vi "Query.vi"(7 "Module Settings":T1(array[cluster]), 8 "error in (no error)":errorcluster, 9 "Region":dbl, 10 "Tray":dbl, 11 "Database Assembly in":refnum<class "Database Assembly.lvclass">) -> (0 "error out":errorcluster, 3 "Database Assembly out":refnum<class "Database Assembly.lvclass">)   [LabVIEW 2018, in "Database Assembly.lvclass"]
uses:
  Database Assembly.lvclass
  Module/Module.lvclass
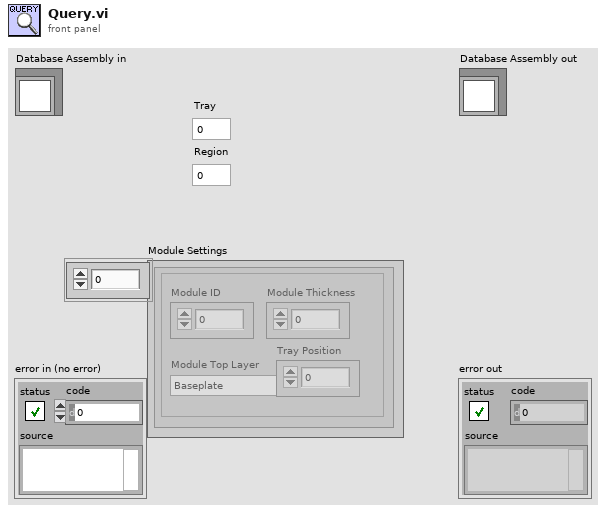
[diagram p1: front panel]
types:
  T1 = cluster{"Module ID":dbl, "Module Thickness":dbl, "Module Top Layer":enum16{"Baseplate", "Kapton", "Sensor", "PCB"}, "Tray Position":dbl}[]
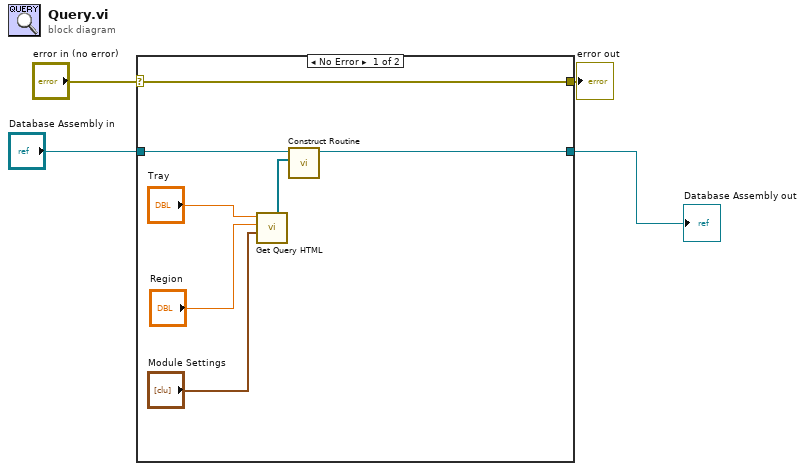
[diagram p0: block diagram]
diagram:
  n1 = case shown="No Error" "error in (no error)" {
    selector: "error in (no error)" -> [w11 w13]
    tunnel: [w11 w13] -> w3
    tunnel: [w10 w12] -> w1
    tunnel: "Database Assembly in" -> [w6 w12]
    frame No Error {
      n2 = call "Get Query HTML.vi"("Module Settings"="Module Settings", "Assembly Tray Region"="Region", "Tray"="Tray") -> ("Module Array"=w7:refnum<class "Module.lvclass">[])  [unwired: 8 in]
      n3 = call "Construct Routine.vi"("Modules"=w7, "Database Assembly in"=w6) -> ("Database Assembly out"=w10:refnum<class "Database Assembly.lvclass">)  [unwired: 8 in, 1 out]
    }
    frame Error {
    }
  }
  "error out" <- w3
  "Database Assembly out" <- w1
